vi "DAQ_D_23.vi"() -> ()   [LabVIEW 2018]
panel:
  out "Digital Waveform Graph":digitalwaveform[](graph)
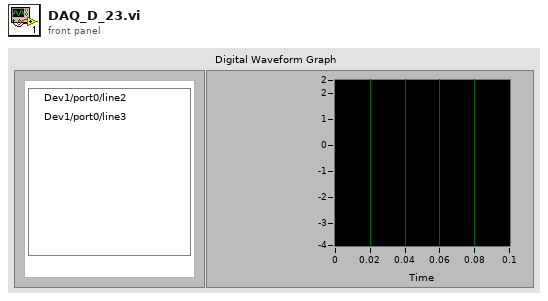
[diagram p1: front panel]
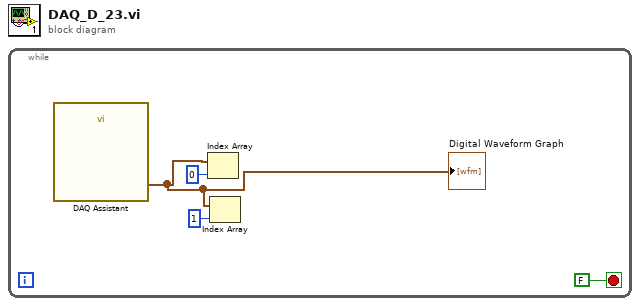
[diagram p0: block diagram]
diagram:
  n1 = while {
    stop <- FALSE stop-if-true
    n2 = call "DAQ Assistant"() -> ("data"=w2:digitalwaveform[])  [unwired: 17 in, 2 out]
    "Digital Waveform Graph" <- w2
    n3 = Index Array(array=w2, index=0) -> ()  [unwired: 1 out]
    n4 = Index Array(array=w2, index=1) -> ()  [unwired: 1 out]
  }
